vi "H3C psw cable 28G QSFP+读写操作.vi"(6 "input_psw":u8[](array[numeric]) format="%.0x", 8 "input_data":u8[](array[numeric]) format="%.0x", 9 "input_mode":string(combo), 10 "Channel":u8 max=5 step=1, 11 "VISA":refnum<visa-resource-name>="COM6") -> (0 "123equal0?":bool, 1 "result":bool, 2 "message":string, 3 "data read":u8[](array[numeric]) format="%.0x")   [LabVIEW 2011]
uses:
  <vilib>/Utility/file.llb/Read From Spreadsheet File (string).vi
panel:
  in  "路径":path
  out "page3 128 Bytes":u8[](array[numeric]) format="%.0x"
  out "page2 128 Bytes":u8[](array[numeric]) format="%.0x"
  out "page1 128 Bytes":u8[](array[numeric]) format="%.0x"
  in  "address":u8
  # "非0page"
  # "这下面全是为0page"
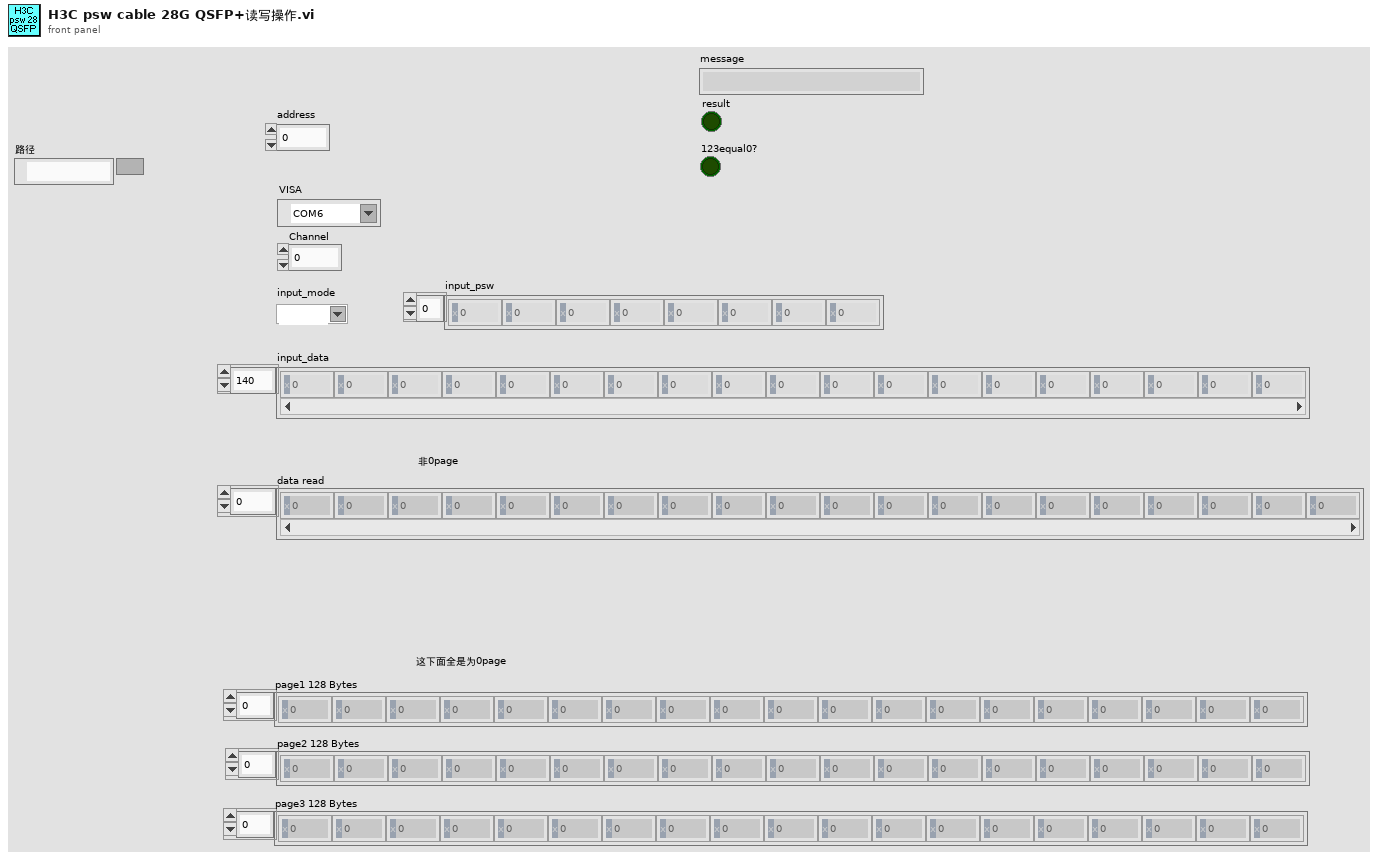
[diagram p1: front panel]
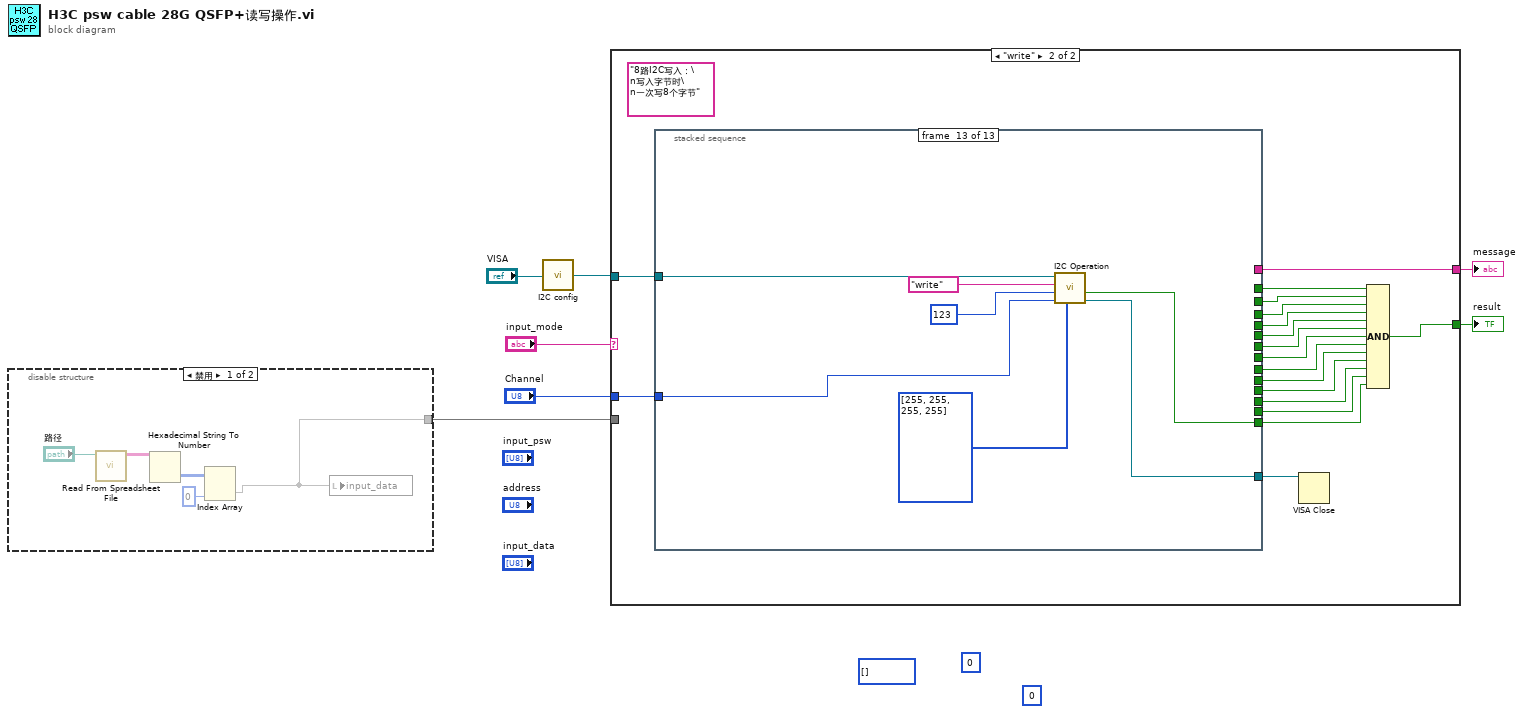
[diagram p0: block diagram]
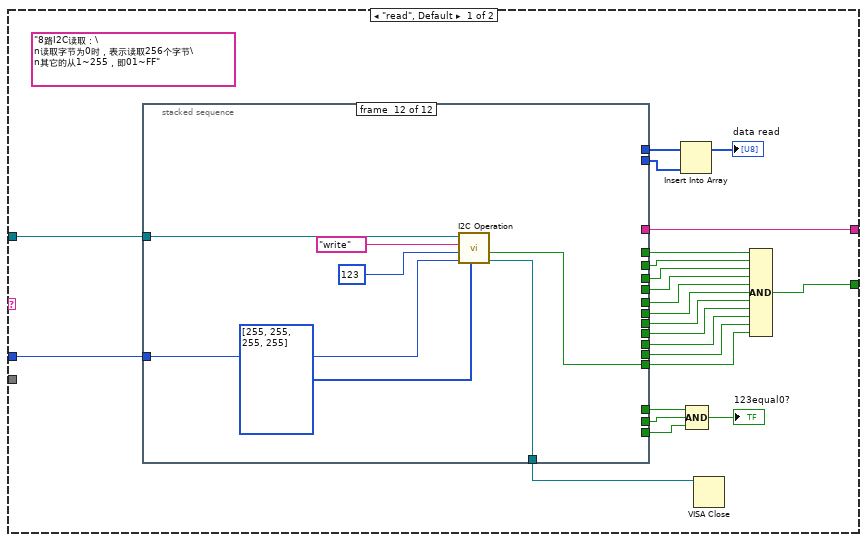
[diagram p3: hidden frame]
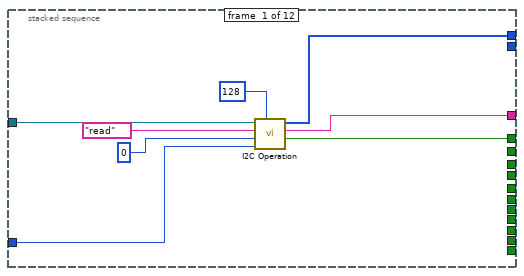
[diagram p4: hidden frame]
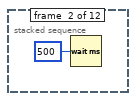
[diagram p5: hidden frame]
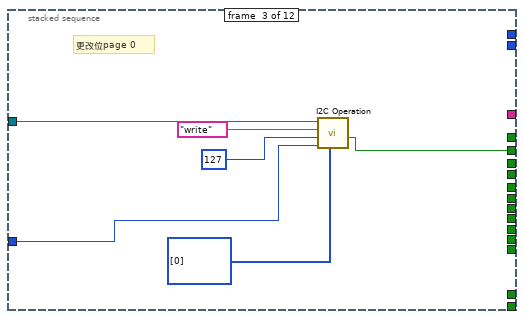
[diagram p6: hidden frame]
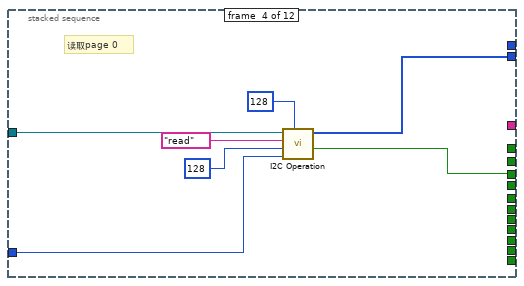
[diagram p7: hidden frame]
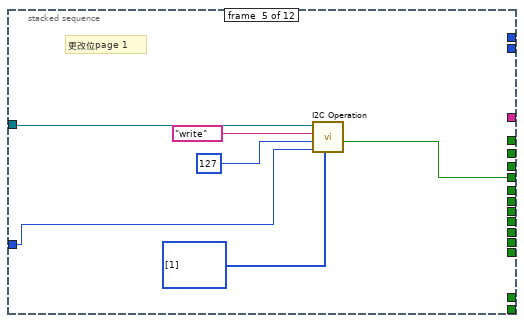
[diagram p8: hidden frame]
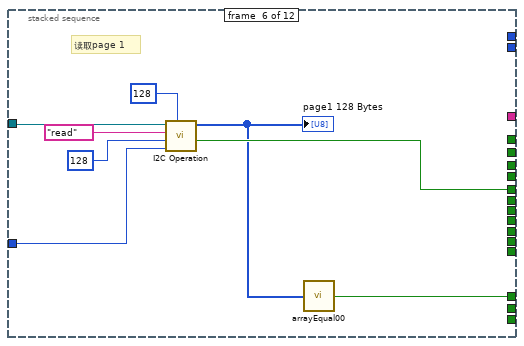
[diagram p9: hidden frame]
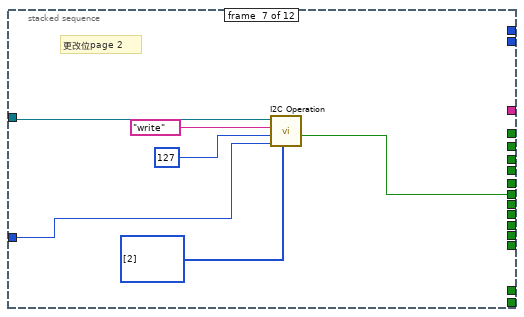
[diagram p10: hidden frame]
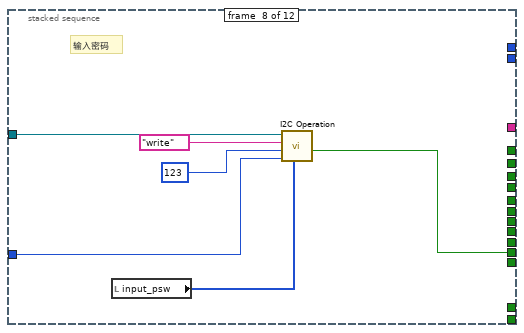
[diagram p11: hidden frame]
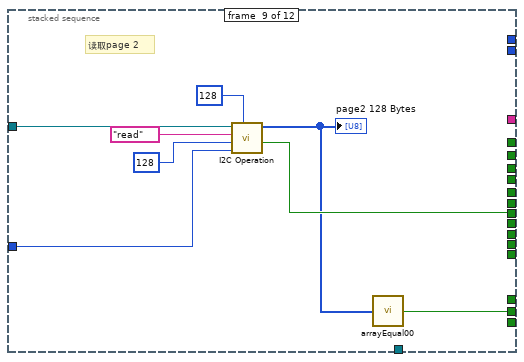
[diagram p12: hidden frame]
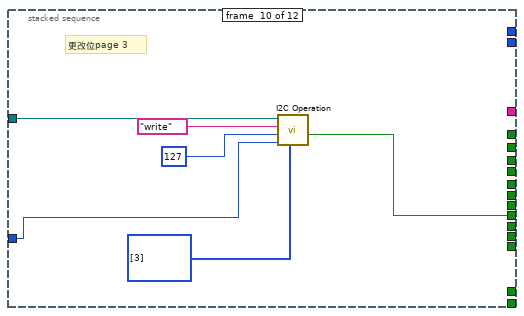
[diagram p13: hidden frame]
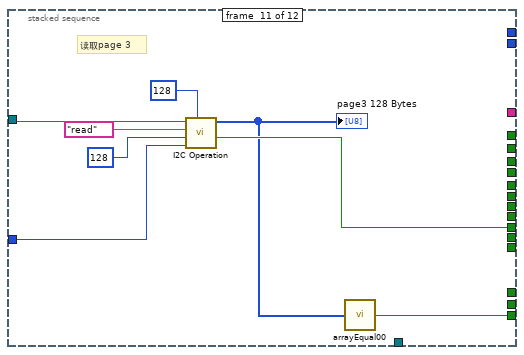
[diagram p14: hidden frame]
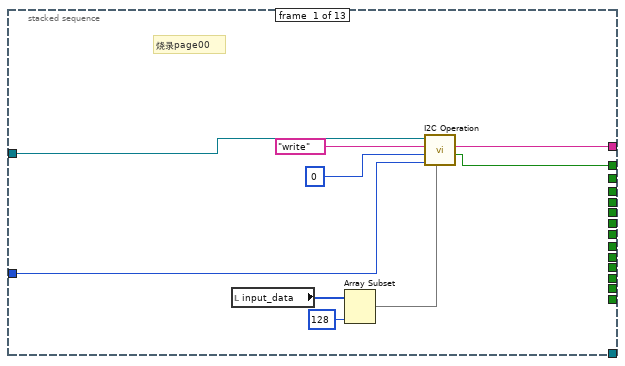
[diagram p15: hidden frame]
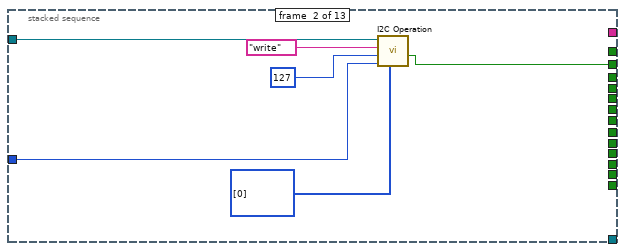
[diagram p16: hidden frame]
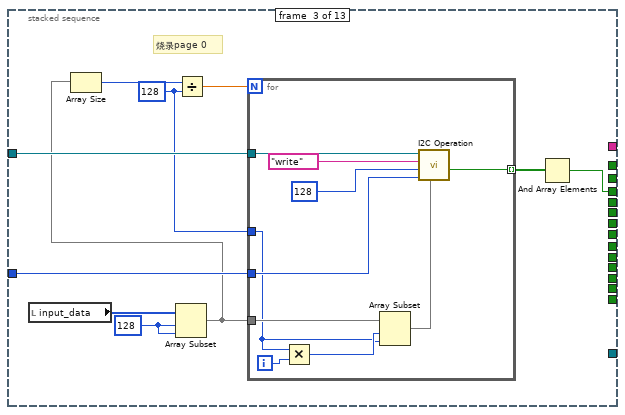
[diagram p17: hidden frame]
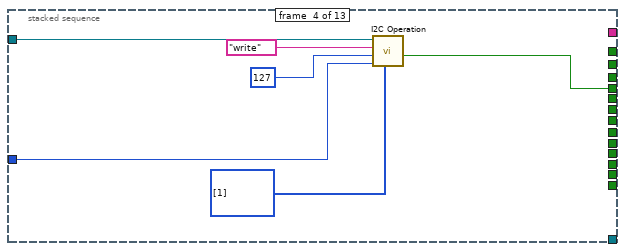
[diagram p18: hidden frame]
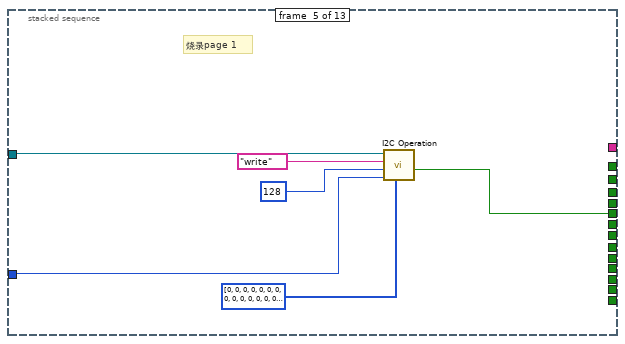
[diagram p19: hidden frame]
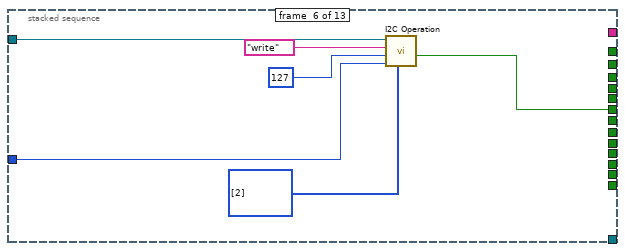
[diagram p20: hidden frame]
diagram:
  (unwired) u8[] []
  (unwired) u8 0
  (unwired) u8 0
  n1 = disable-structure shown="禁用" {
    disable-tunnel: [w8 _] -> w3
    frame Disabled {
      n2 = call-poly <vilib>:"Read From Spreadsheet File.vi"("file path (dialog if empty)"="路径") -> ("all rows"=w11:string[][])  [unwired: 6 in, 4 out]
      n3 = Hexadecimal String To Number(string=w11) -> (number=w10:u32[][])  [unwired: 2 in, 1 out]
      n4 = Index Array(array=w10, index (col)=0 ("禁用的索引 (列)")) -> (element=w8:u32[])  [unwired: 1 in]
      n5 = local write "input_data"(w8) -> ()
    }
    frame Enabled {
    }
  }
  n6 = call "I2C config.vi"("VISA"="VISA") -> ("VISA资源名称输出"=w1:refnum<visa-resource-name>)
  n7 = case shown="\"write\"" "input_mode" {
    tunnel: w1 -> [w35 w130]
    tunnel: "Channel" -> [w34 w129]
    tunnel: [w33 w128] -> w5
    tunnel: [w20 w114] -> w4
    tunnel: w3 -> [_ _]
    frame "read", Default {
      (unwired) "8路I2C读取：\n读取字节为0时，表示读取256个字节\n其它的从1~255，即01~FF"
      n8 = stacked-sequence {
        tunnel: w35 -> [w43 _ w47 w57 w60 w68 w74 w80 w88 w94 w102 w110]
        tunnel: w34 -> [w39 _ w46 w53 w59 w67 w73 w79 w87 w93 w101 w109]
        tunnel: [w38 _ _ _ _ _ _ _ _ _ _ _] -> w33
        tunnel: [w37 _ _ _ _ _ _ _ _ _ _ _] -> w29
        tunnel: [w36 _ _ _ _ _ _ _ _ _ _ _] -> w32
        tunnel: [_ _ _ w52 _ _ _ _ _ _ _ _] -> w31
        tunnel: [_ _ w45 _ _ _ _ _ _ _ _ _] -> w28
        tunnel: [_ _ _ w51 _ _ _ _ _ _ _ _] -> w27
        tunnel: [_ _ _ _ w58 _ _ _ _ _ _ _] -> w26
        tunnel: [_ _ _ _ _ w66 _ _ _ _ _ _] -> w25
        tunnel: [_ _ _ _ _ _ w72 _ _ _ _ _] -> w24
        tunnel: [_ _ _ _ _ _ _ _ w86 _ _ _] -> w23
        tunnel: [_ _ _ _ _ _ _ _ _ w92 _ _] -> w22
        tunnel: [_ _ _ _ _ _ _ _ _ _ w100 _] -> w21
        tunnel: [_ _ _ _ _ _ _ w78 _ _ _ _] -> w19
        tunnel: [_ _ _ _ _ _ _ _ _ _ _ w107] -> w18
        tunnel: [_ _ _ _ _ w64 _ _ _ _ _ _] -> w17
        tunnel: [_ _ _ _ _ _ _ _ w85 _ _ _] -> w16
        tunnel: [_ _ _ _ _ _ _ _ _ _ w99 _] -> w15
        tunnel: [_ _ _ _ _ _ _ _ _ _ _ w106] -> w13
        frame #0 {
          n9 = call "I2C Operation.vi"("size"=128, "Channel"=w39, "address"=u8 0, "mode"="read", "VISA"=w43) -> ("result"=w37:bool, "message"=w38:string, "Data Out"=w36:u8[])  [unwired: 3 in, 1 out]
        }
        frame #1 {
          n10 = Wait (ms)(milliseconds to wait=u32 500 ("等待时间（毫秒）")) -> ()  [unwired: 1 out]
        }
        frame #2 {
          # "更改位page 0"
          n11 = call "I2C Operation.vi"("input_data"=u8[] [0], "Channel"=w46, "address"=u8 127, "mode"="write", "VISA"=w47) -> ("result"=w45:bool)  [unwired: 3 in, 3 out]
        }
        frame #3 {
          # "读取page 0"
          n12 = call "I2C Operation.vi"("size"=128, "Channel"=w53, "address"=u8 128, "mode"="read", "VISA"=w57) -> ("result"=w51:bool, "Data Out"=w52:u8[])  [unwired: 3 in, 2 out]
        }
        frame #4 {
          # "更改位page 1"
          n13 = call "I2C Operation.vi"("input_data"=u8[] [1], "Channel"=w59, "address"=u8 127, "mode"="write", "VISA"=w60) -> ("result"=w58:bool)  [unwired: 3 in, 3 out]
        }
        frame #5 {
          # "读取page 1"
          n14 = call "I2C Operation.vi"("size"=128, "Channel"=w67, "address"=u8 128, "mode"="read", "VISA"=w68) -> ("result"=w66:bool, "Data Out"=w65:u8[])  [unwired: 3 in, 2 out]
          "page1 128 Bytes" <- w65
          n15 = call "arrayEqual00.vi"("input"=w65) -> ("equal"=w64:bool)
        }
        frame #6 {
          # "更改位page 2"
          n16 = call "I2C Operation.vi"("input_data"=u8[] [2], "Channel"=w73, "address"=u8 127, "mode"="write", "VISA"=w74) -> ("result"=w72:bool)  [unwired: 3 in, 3 out]
        }
        frame #7 {
          # "输入密码"
          n17 = local read "input_psw"() -> (w81:u8[])
          n18 = call "I2C Operation.vi"("input_data"=w81, "Channel"=w79, "address"=u8 123, "mode"="write", "VISA"=w80) -> ("result"=w78:bool)  [unwired: 3 in, 3 out]
        }
        frame #8 {
          # "读取page 2"
          n19 = call "I2C Operation.vi"("size"=128, "Channel"=w87, "address"=u8 128, "mode"="read", "VISA"=w88) -> ("result"=w86:bool, "Data Out"=w84:u8[])  [unwired: 3 in, 2 out]
          "page2 128 Bytes" <- w84
          n20 = call "arrayEqual00.vi"("input"=w84) -> ("equal"=w85:bool)
        }
        frame #9 {
          # "更改位page 3"
          n21 = call "I2C Operation.vi"("input_data"=u8[] [3], "Channel"=w93, "address"=u8 127, "mode"="write", "VISA"=w94) -> ("result"=w92:bool)  [unwired: 3 in, 3 out]
        }
        frame #10 {
          # "读取page 3"
          n22 = call "I2C Operation.vi"("size"=128, "Channel"=w101, "address"=u8 128, "mode"="read", "VISA"=w102) -> ("result"=w100:bool, "Data Out"=w98:u8[])  [unwired: 3 in, 2 out]
          "page3 128 Bytes" <- w98
          n23 = call "arrayEqual00.vi"("input"=w98) -> ("equal"=w99:bool)
        }
        frame #11 {
          n24 = call "I2C Operation.vi"("input_data"=u8[] [255, 255, 255, 255], "Channel"=w109, "address"=u8 123, "mode"="write", "VISA"=w110) -> ("VISA  2"=w106:refnum<visa-resource-name>, "result"=w107:bool)  [unwired: 3 in, 2 out]
        }
      }
      n25 = Insert Into Array(array=w32, new element=w31) -> (→"data read":u8[])  [unwired: 1 in]
      n26 = Compound Arithmetic op=AND(w17, w16, w15) -> (→"123equal0?":bool)
      n27 = VISA Close(VISA resource name=w13) -> ()  [unwired: 1 in, 1 out]
      n28 = Compound Arithmetic op=AND(w29, w28, w27, w26, w25, w24, w23, w22, w21, w19, w18) -> (w20:bool)
    }
    frame "write" {
      (unwired) "8路I2C写入：\n写入字节时\n一次写8个字节"
      n29 = stacked-sequence {
        tunnel: w130 -> [w139 w145 w155 w167 w174 w180 w186 w192 w197 w204 w211 w217 w224]
        tunnel: w129 -> [w137 w143 w154 w168 w173 w181 w187 w191 w198 w203 w210 w216 w223]
        tunnel: [w136 _ _ _ _ _ _ _ _ _ _ _ _] -> w128
        tunnel: [w135 _ _ _ _ _ _ _ _ _ _ _ _] -> w127
        tunnel: [_ w140 _ _ _ _ _ _ _ _ _ _ _] -> w126
        tunnel: [_ _ w146 _ _ _ _ _ _ _ _ _ _] -> w125
        tunnel: [_ _ _ w166 _ _ _ _ _ _ _ _ _] -> w124
        tunnel: [_ _ _ _ w172 _ _ _ _ _ _ _ _] -> w123
        tunnel: [_ _ _ _ _ w178 _ _ _ _ _ _ _] -> w122
        tunnel: [_ _ _ _ _ _ w184 _ _ _ _ _ _] -> w121
        tunnel: [_ _ _ _ _ _ _ w190 _ _ _ _ _] -> w120
        tunnel: [_ _ _ _ _ _ _ _ w196 _ _ _ _] -> w119
        tunnel: [_ _ _ _ _ _ _ _ _ w202 _ _ _] -> w118
        tunnel: [_ _ _ _ _ _ _ _ _ _ w208 _ _] -> w117
        tunnel: [_ _ _ _ _ _ _ _ _ _ _ w214 _] -> w116
        tunnel: [_ _ _ _ _ _ _ _ _ _ _ _ w221] -> w115
        tunnel: [_ _ _ _ _ _ _ _ _ _ _ _ w220] -> w113
        frame #0 {
          # "烧录page00"
          n30 = local read "input_data"() -> (w133:u8[])
          n31 = Array Subset(array=w133, length=128 ("长度")) -> (w131:u8[])  [unwired: 1 in]
          n32 = call "I2C Operation.vi"("input_data"=w131, "Channel"=w137, "address"=u8 0, "mode"="write", "VISA"=w139) -> ("result"=w135:bool, "message"=w136:string)  [unwired: 3 in, 2 out]
        }
        frame #1 {
          n33 = call "I2C Operation.vi"("input_data"=u8[] [0], "Channel"=w143, "address"=u8 127, "mode"="write", "VISA"=w145) -> ("result"=w140:bool)  [unwired: 3 in, 3 out]
        }
        frame #2 {
          w148 = 128 ("y")
          w152 = 128 ("索引")
          # "烧录page 0"
          n34 = local read "input_data"() -> (w153:u8[])
          n35 = Array Subset(array=w153, index=w152, length=w152) -> (w151:u8[])
          n36 = Array Size(array=w151) -> (size(s)=w150:i32)
          n37 = Divide(x=w150, y=w148) -> (x/y=w149:dbl)
          n38 = for {
            N: w149 -> [_]
            tunnel: w155 -> [w165]
            tunnel: w154 -> [w163]
            tunnel: [w161] -> w147 mode=indexing
            tunnel: w151 -> [w160]
            tunnel: w148 -> [w157]
            i -> [w159]
            n39 = Multiply(x=w157, y=w159) -> (x*y=w158:i32)
            n40 = Array Subset(array=w160, index=w158, length=w157) -> (w156:u8[])
            n41 = call "I2C Operation.vi"("input_data"=w156, "Channel"=w163, "address"=u8 128, "mode"="write", "VISA"=w165) -> ("result"=w161:bool)  [unwired: 3 in, 3 out]
          }
          n42 = And Array Elements(Boolean array=w147) -> (logical AND=w146:bool)
        }
        frame #3 {
          n43 = call "I2C Operation.vi"("input_data"=u8[] [1], "Channel"=w168, "address"=u8 127, "mode"="write", "VISA"=w167) -> ("result"=w166:bool)  [unwired: 3 in, 3 out]
        }
        frame #4 {
          # "烧录page 1"
          n44 = call "I2C Operation.vi"("input_data"=u8[] [0, 0, 0, 0, 0, 0, 0, 0, 0, 0, 0, 0, 0, 0, 0, 0, 0, 0, 0, 0, 0, 0, 0, 0, 0, 0, 0, 0, 0, 0, 0, 0, 0, 0, 0, 0, 0, 0, 0, 0, 0, 0, 0, 0, 0, 0, 0, 0, 0, 0, 0, 0, 0, 0, 0, 0, 0, 0, 0, 0, 0, 0, 0, 0, 0, 0, 0, 0, 0, 0, 0, 0, 0, 0, 0, 0, 0, 0, 0, 0, 0, 0, 0, 0, 0, 0, 0, 0, 0, 0, 0, 0, 0, 0, 0, 0, 0, 0, 0, 0, 0, 0, 0, 0, 0, 0, 0, 0, 0, 0, 0, 0, 0, 0, 0, 0, 0, 0, 0, 0, 0, 0, 0, 0, 0, 0, 0, 0], "Channel"=w173, "address"=u8 128, "mode"="write", "VISA"=w174) -> ("result"=w172:bool)  [unwired: 3 in, 3 out]
        }
        frame #5 {
          n45 = call "I2C Operation.vi"("input_data"=u8[] [2], "Channel"=w181, "address"=u8 127, "mode"="write", "VISA"=w180) -> ("result"=w178:bool)  [unwired: 3 in, 3 out]
        }
        frame #6 {
          n46 = local read "input_psw"() -> (w185:u8[])
          n47 = call "I2C Operation.vi"("input_data"=w185, "Channel"=w187, "address"=u8 123, "mode"="write", "VISA"=w186) -> ("result"=w184:bool)  [unwired: 3 in, 3 out]
        }
        frame #7 {
          # "烧录page 2"
          n48 = call "I2C Operation.vi"("input_data"=u8[] [0, 0, 0, 0, 0, 0, 0, 0, 0, 0, 0, 0, 0, 0, 0, 0, 0, 0, 0, 0, 0, 0, 0, 0, 0, 0, 0, 0, 0, 0, 0, 0, 0, 0, 0, 0, 0, 0, 0, 0, 0, 0, 0, 0, 0, 0, 0, 0, 0, 0, 0, 0, 0, 0, 0, 0, 0, 0, 0, 0, 0, 0, 0, 0, 0, 0, 0, 0, 0, 0, 0, 0, 0, 0, 0, 0, 0, 0, 0, 0, 0, 0, 0, 0, 0, 0, 0, 0, 0, 0, 0, 0, 0, 0, 0, 0, 0, 0, 0, 0, 0, 0, 0, 0, 0, 0, 0, 0, 0, 0, 0, 0, 0, 0, 0, 0, 0, 0, 0, 0, 0, 0, 0, 0, 0, 0, 0, 0], "Channel"=w191, "address"=u8 128, "mode"="write", "VISA"=w192) -> ("result"=w190:bool)  [unwired: 3 in, 3 out]
        }
        frame #8 {
          n49 = call "I2C Operation.vi"("input_data"=u8[] [3], "Channel"=w198, "address"=u8 127, "mode"="write", "VISA"=w197) -> ("result"=w196:bool)  [unwired: 3 in, 3 out]
        }
        frame #9 {
          # "烧录page 3"
          n50 = call "I2C Operation.vi"("input_data"=u8[] [0, 0, 0, 0, 0, 0, 0, 0, 0, 0, 0, 0, 0, 0, 0, 0, 0, 0, 0, 0, 0, 0, 0, 0, 0, 0, 0, 0, 0, 0, 0, 0, 0, 0, 0, 0, 0, 0, 0, 0, 0, 0, 0, 0, 0, 0, 0, 0, 0, 0, 0, 0, 0, 0, 0, 0, 0, 0, 0, 0, 0, 0, 0, 0, 0, 0, 0, 0, 0, 0, 0, 0, 0, 0, 0, 0, 0, 0, 0, 0, 0, 0, 0, 0, 0, 0, 0, 0, 0, 0, 0, 0, 0, 0, 0, 0, 0, 0, 0, 0, 0, 0, 0, 0, 0, 0, 0, 0, 0, 0, 0, 0, 0, 0, 0, 0, 0, 0, 0, 0, 0, 0, 0, 0, 0, 0, 0, 0], "Channel"=w203, "address"=u8 128, "mode"="write", "VISA"=w204) -> ("result"=w202:bool)  [unwired: 3 in, 3 out]
        }
        frame #10 {
          n51 = call "I2C Operation.vi"("input_data"=u8[] [0], "Channel"=w210, "address"=u8 127, "mode"="write", "VISA"=w211) -> ("result"=w208:bool)  [unwired: 3 in, 3 out]
        }
        frame #11 {
          n52 = call "I2C Operation.vi"("input_data"=u8[] [226, 23, 130, 37], "Channel"=w216, "address"=u8 123, "mode"="write", "VISA"=w217) -> ("result"=w214:bool)  [unwired: 3 in, 3 out]
        }
        frame #12 {
          n53 = call "I2C Operation.vi"("input_data"=u8[] [255, 255, 255, 255], "Channel"=w223, "address"=u8 123, "mode"="write", "VISA"=w224) -> ("VISA  2"=w220:refnum<visa-resource-name>, "result"=w221:bool)  [unwired: 3 in, 2 out]
        }
      }
      n54 = VISA Close(VISA resource name=w113) -> ()  [unwired: 1 in, 1 out]
      n55 = Compound Arithmetic op=AND(w127, w126, w125, w124, w123, w122, w121, w120, w119, w118, w117, w116, w115) -> (w114:bool)
    }
  }
  "message" <- w5
  "result" <- w4
